vi "Day 05 (Part Two).vi"() -> ()   [LabVIEW 2021]
panel:
  out "result":u32
  # "VI will run approx. for 30 minutes to get the result and requires x64 version of LabVIEW!"
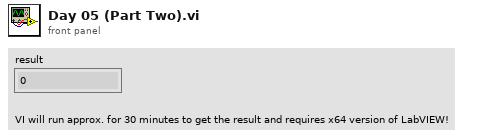
[diagram p1: front panel]
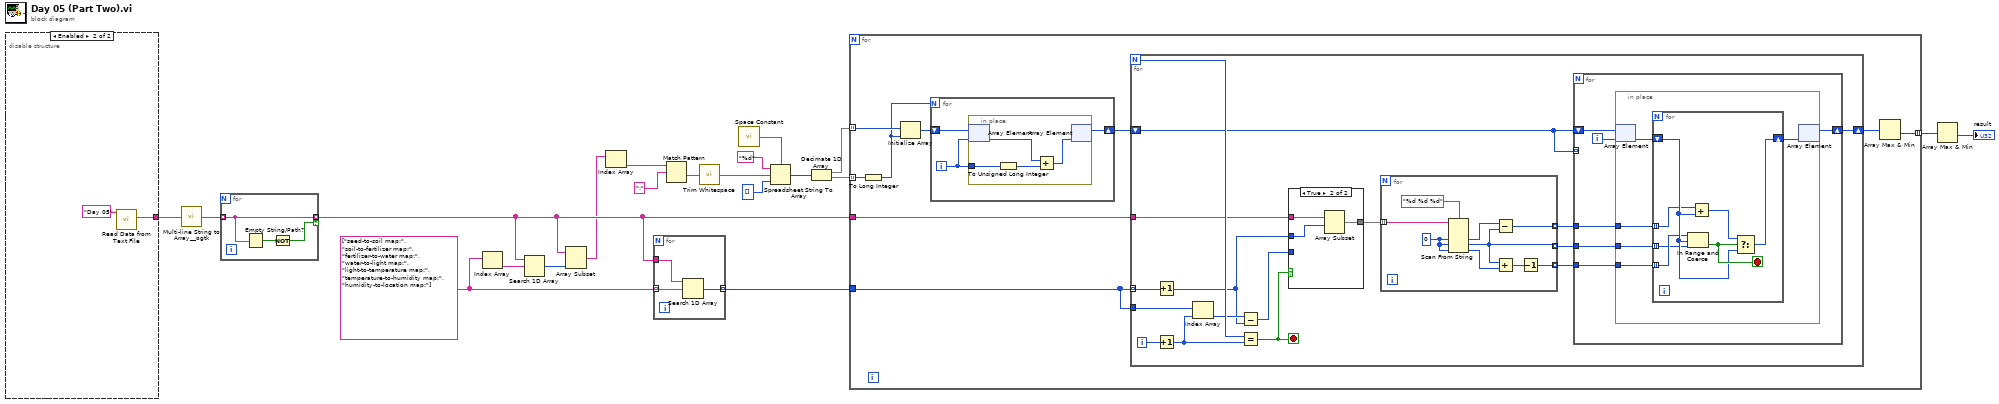
[diagram p0: block diagram]
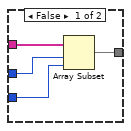
[diagram p2: hidden frame]
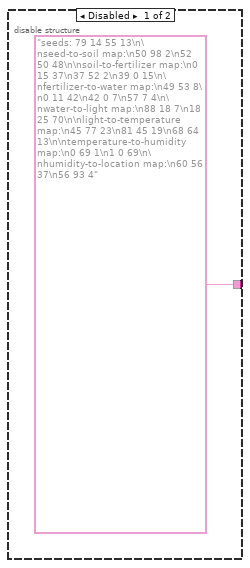
[diagram p3: hidden frame]
diagram:
  w17 = string[] ["seed-to-soil map:", "soil-to-fertilizer map:", "fertilizer-to-water map:", "water-to-light map:", "light-to-temperature map:", "temperature-to-humidity map:", "humidity-to-location map:"]
  n1 = disable-structure shown="Enabled" {
    disable-tunnel: ["seeds: 79 14 55 13\n\nseed-to-soil map:\n50 98 2\n52 50 48\n\nsoil-to-fertilizer map:\n0 15 37\n37 52 2\n39 0 15\n\nfertilizer-to-water map:\n49 53 8\n0 11 42\n42 0 7\n57 7 4\n\nwater-to-light map:\n88 18 7\n18 25 70\n\nlight-to-temperature map:\n45 77 23\n81 45 19\n68 64 13\n\ntemperature-to-humidity map:\n0 69 1\n1 0 69\n\nhumidity-to-location map:\n60 56 37\n56 93 4" w23] -> w20
    frame Disabled {
    }
    frame Enabled {
      n2 = call "Read Data from Text File.vi"("Subfolder"="Day 05") -> ("data"=w23:string)  [unwired: 10 in]
    }
  }
  n3 = call <userlib>:"Multi-line String to Array__ogtk.vi"("string"=w20) -> ("lines"=w15:string[])
  n4 = for {
    tunnel: w15 -> [w25] mode=indexing
    tunnel: [w25] -> w14 mode=indexing if=w24
    n5 = Empty String/Path?(string/path=w25) -> (empty?=w26:bool)
    n6 = Not(x=w26) -> (.not. x?=w24:bool)
  }
  n7 = Index Array(array=w17) -> (element=w19:string)  [unwired: 1 in]
  n8 = Search 1D Array(1D array=w14, element=w19) -> (index of element=w18:i32)  [unwired: 1 in]
  n9 = Array Subset(array=w14, length=w18) -> (w13:string[])  [unwired: 1 in]
  n10 = Index Array(array=w13) -> (element=w12:string)  [unwired: 1 in]
  n11 = for {
    tunnel: w17 -> [w29] mode=indexing
    tunnel: [w28] -> w16 mode=indexing
    tunnel: w14 -> [w27]
    n12 = Search 1D Array(1D array=w27, element=w29) -> (index of element=w28:i32)  [unwired: 1 in]
  }
  n13 = Match Pattern(string=w12, regular expression=":") -> (after substring=w10:string)  [unwired: 1 in, 3 out]
  n14 = call <vilib>:"Trim Whitespace.vi"("string"=w10) -> ("trimmed string"=w9:string)  [unwired: 1 in]
  n15 = call <vilib>:"Space Constant.vi"() -> ("String"=w7:string)
  n16 = Spreadsheet String To Array(delimiter (Tab)=w7, format string="%d", spreadsheet string=w9, array type (2D Dbl)=u32[] []) -> (array=w4:u32[])
  n17 = Decimate 1D Array(w4) -> (w3:u32[], w2:u32[])
  n18 = for {
    tunnel: w16 -> [w38]
    tunnel: w14 -> [w37]
    tunnel: [w30] -> w1 mode=indexing
    tunnel: w3 -> [w35] mode=indexing
    tunnel: w2 -> [w34] mode=indexing
    n19 = To Long Integer(number=w34) -> (32bit integer=w32:i32)
    n20 = Initialize Array(w35, w32) -> (w33:u32[])
    n21 = for {
      N: w32 -> [_]
      shift-right: [w39] -> w36
      shift-left: w33 -> [w41]
      i -> [w40]
      n22 = in-place {
        in-place-border: w40 -> [w44]
        n23 = in-place-array #1(w41, w40) -> (w45:u32)
        n24 = To Unsigned Long Integer(number=w44) -> (unsigned 32bit integer=w43:u32)
        n25 = Add(x=w45, y=w43) -> (x+y=w42:u32)
        n26 = in-place-array #1(w42) -> (w39:u32[])  [unwired: 1 out]
      }
    }
    n27 = for {
      N -> [w59]
      tunnel: w38 -> [w55] mode=indexing
      tunnel: w38 -> [w61]
      tunnel: w37 -> [w58]
      shift-right: [w52] -> w31
      shift-left: w36 -> [w46]
      i -> [w51]
      stop <- w54 stop-if-true
      n28 = Increment(x=w55) -> (x+1=w53:i32)
      n29 = Increment(x=w51) -> (x+1=w60:i32)
      n30 = Index Array(array=w61, index=w60) -> (element=w57:i32)
      n31 = Subtract(x=w57, y=w53) -> (x-y=w56:i32)
      n32 = Equal?(x=w59, y=w60) -> (x = y?=w54:bool)
      n33 = case shown="True" w54 {
        tunnel: w58 -> [w74 w77]
        tunnel: w56 -> [w73 _]
        tunnel: w53 -> [w72 w75]
        tunnel: [w71 w76] -> w50
        frame False {
          n34 = Array Subset(array=w74, index=w72, length=w73) -> (w71:string[])
        }
        frame True {
          n35 = Array Subset(array=w77, index=w75) -> (w76:string[])  [unwired: 1 in]
        }
      }
      n36 = for {
        tunnel: w50 -> [w69] mode=indexing
        tunnel: [w64] -> w49 mode=indexing
        tunnel: [w63] -> w48 mode=indexing
        tunnel: [w65] -> w47 mode=indexing
        w70 = u32 0 ("default value 1")
        n37 = Scan From String(format string="%d %d %d", input string=w69, default 1=w70, default 2=w70, default 3=w70) -> (output 1=w62:u32, output 2=w63:u32, output 3=w67:u32)  [unwired: 2 in, 3 out]
        n38 = Subtract(x=w62, y=w63) -> (x-y=w64:u32)
        n39 = Add(x=w63, y=w67) -> (x+y=w66:u32)
        n40 = Decrement(x=w66) -> (x-1=w65:u32)
      }
      n41 = for {
        shift-right: [w81] -> w52
        shift-left: w46 -> [w83]
        tunnel: w49 -> [w80]
        tunnel: w48 -> [w79]
        tunnel: w47 -> [w78]
        tunnel: w46 -> [_] mode=indexing
        i -> [w82]
        n42 = in-place {
          in-place-border: w80 -> [w86]
          in-place-border: w79 -> [w85]
          in-place-border: w78 -> [w84]
          n43 = in-place-array #2(w83, w82) -> (w87:u32)
          n44 = for {
            shift-right: [w93] -> w88
            shift-left: w87 -> [w92]
            tunnel: w86 -> [w90] mode=indexing
            tunnel: w85 -> [w89] mode=indexing
            tunnel: w84 -> [w91] mode=indexing
            stop <- w95 stop-if-true
            n45 = In Range and Coerce(upper limit=w91, x=w92, lower limit=w89) -> (In Range?=w95:bool)  [unwired: 1 out]
            n46 = Add(x=w90, y=w92) -> (x+y=w94:u32)
            n47 = Select(t=w94, s=w95, f=w92) -> (s? t:f=w93:u32)
          }
          n48 = in-place-array #2(w88) -> (w81:u32[])  [unwired: 1 out]
        }
      }
    }
    n49 = Array Max & Min(array=w31) -> (min value=w30:u32)  [unwired: 3 out]
  }
  n50 = Array Max & Min(array=w1) -> (min value=→"result":u32)  [unwired: 3 out]
